vi "CRYWindow Activeing.vi"(9 "nID":i32, 10 "ActiveTF":bool) -> ()   [LabVIEW 2013]
uses:
  CRYMain Sub Window Global.vi
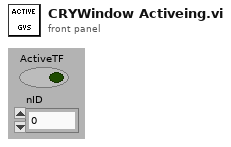
[diagram p1: front panel]
types:
  T1 = typedef "LVRectTypeDef.ctl" = cluster{"Left":i16, "Top":i16, "Right":i16, "Bottom":i16}
  T2 = cluster{"nType":i32, "nParent":i32, "pVIW":refnum<vi>, "pSPW":refnum<vi>, "nTypeF":i32, "pVIF":refnum<vi>, "pSPF":refnum<vi>, "nIDSpliter":i32, "nProperty":i32, "Bound":T1, "nID":i32, "nData":i32, "sData":string, "pWVI":refnum<vi>, "sTitle":string, "cPages":cluster{"nPage":i32, "sTitle":string, "sIcon":string, "pVI":refnum<vi>, "nID":i32}[], "pTab":refnum<vi>, "nIDPages":i32[], "pSPT":refnum<vi>, "sTemp":string, "nDockID":i32, "nDockLR":i32, "sIcon":string}
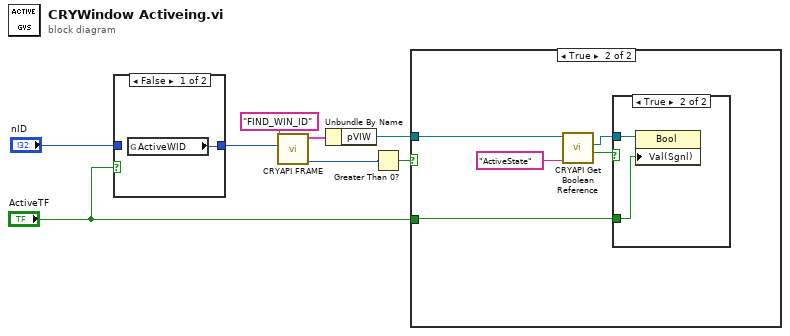
[diagram p0: block diagram]
diagram:
  n1 = case shown="False" "ActiveTF" {
    tunnel: "nID" -> [_ w10]
    tunnel: [w9 w10] -> w1
    frame False {
      n2 = global read "CRYMain Sub Window Global.vi" "ActiveWID"() -> (w9:i32)
    }
    frame True {
    }
  }
  n3 = call "CRYAPI FRAME.vi"("nData"=w1, "sAction"="FIND_WIN_ID") -> ("nData_Out"=w5:i32, "tFrame_Out"=w8:T2)  [unwired: 6 in, 2 out]
  n4 = Unbundle By Name(w8) -> ("pVIW"=w4:refnum<vi>)
  n5 = Greater Than 0?(x=w5) -> (x > 0?=w6:bool)
  n6 = case shown="True" w6 {
    tunnel: w4 -> [_ w15]
    tunnel: "ActiveTF" -> [_ w11]
    frame False {
    }
    frame True {
      n7 = call "CRYAPI Get Boolean Reference.vi"("Label Name"="ActiveState", "VI Refnum"=w15) -> ("Boolean"=w13:bool, "Boolean Ref"=w12:refnum<vi>)  [unwired: 8 out]
      n8 = case shown="True" w13 {
        tunnel: w12 -> [_ w17]
        tunnel: w11 -> [_ w16]
        frame False {
        }
        frame True {
          n9 = property class="Bool"(reference=w17, "Val(Sgnl)"=w16) -> ()  [unwired: 1 in, 2 out]
        }
      }
    }
  }
